vi "过滤数组元素(CTRL-REF).vi"(8 "error in (no error)":errorcluster caption="错误输入（无错误）", 10 "过滤元素":refnum<vi>, 11 "输入数组":refnum<vi>[](array[refnum])) -> (0 "error out":errorcluster caption="错误输出", 2 "已过滤元素索引":i32[](array[numeric]), 3 "输出数组":refnum<vi>[](array[refnum]))   [LabVIEW 2011]
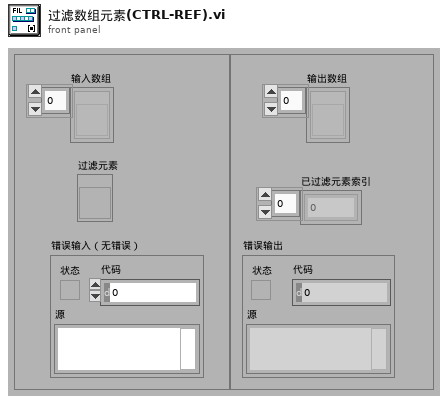
[diagram p1: front panel]
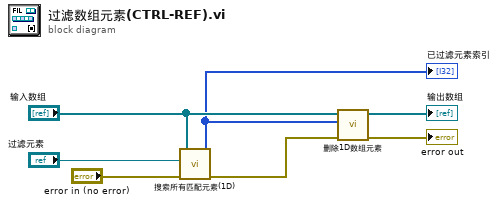
[diagram p0: block diagram]
diagram:
  n1 = call-poly "搜索所有匹配元素(1D).vi"("error in (no error)"="error in (no error)", "元素"="过滤元素", "数组"="输入数组") -> ("error out"=w5:errorcluster, "匹配元素索引"=w1:i32[])  [unwired: 6 in, 1 out]
  "已过滤元素索引" <- w1
  n2 = call-poly "删除1D数组元素.vi"("error in (no error)"=w5, "索引"=w1, "输入数组"="输入数组") -> ("error out"=→"error out":errorcluster, "剩余元素"=→"输出数组":refnum<vi>[])  [unwired: 6 in, 1 out]
